vi "Field Types in Memory.vi"() -> (3 "Creatable Field Types":refnum<class "Type.lvclass">[](array[class]))   [LabVIEW 2020, in "Conditum-Tools.lvlib"]
uses:
  Conditum-Tools.lvlib
  Conditum/Columns/Boolean/Boolean.lvclass
  Conditum/Columns/Double/Double.lvclass
  Conditum/Columns/Integer/Integer.lvclass
  Conditum/Columns/String/String.lvclass
  Conditum/Columns/Text/Text.lvclass
  Conditum/Columns/Timestamp/Timestamp.lvclass
  Conditum/Columns/Relation/Relation.lvclass
  C:/dev/lv20CE/lv-conditum/Conditum/Columns/Type/Type.lvclass
  C:/dev/lv20CE/lv-conditum/Conditum/Columns/Boolean/Boolean.lvclass
  C:/dev/lv20CE/lv-conditum/Conditum/Columns/Double/Double.lvclass
  C:/dev/lv20CE/lv-conditum/Conditum/Columns/Integer/Integer.lvclass
  C:/dev/lv20CE/lv-conditum/Conditum/Columns/Timestamp/Timestamp.lvclass
  C:/dev/lv20CE/lv-conditum/Conditum/Columns/Relation/Relation.lvclass
  C:/dev/lv20CE/lv-conditum/Conditum/Columns/String/String.lvclass
  C:/dev/lv20CE/lv-conditum/Conditum/Columns/Text/Text.lvclass
  Conditum/Columns/Type/Type.lvclass
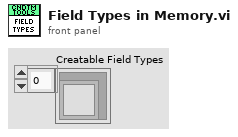
[diagram p1: front panel]
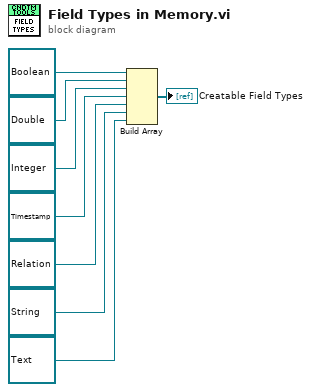
[diagram p0: block diagram]
diagram:
  n1 = Build Array(refnum<class "Boolean.lvclass"> refnum ("Conditum:Columns:Boolean.lvclass"), refnum<class "Double.lvclass"> refnum ("Conditum:Columns:Double.lvclass"), refnum<class "Integer.lvclass"> refnum ("Conditum:Columns:Integer.lvclass"), refnum<class "Timestamp.lvclass"> refnum ("Conditum:Columns:Timestamp.lvclass"), refnum<class "Relation.lvclass"> refnum ("Conditum:Columns:Relation.lvclass"), refnum<class "String.lvclass"> refnum ("Conditum:Columns:String.lvclass"), refnum<class "Text.lvclass"> refnum ("Conditum:Columns:Text.lvclass")) -> (→"Creatable Field Types":refnum<class "Type.lvclass">[])
